vi "SavingToExistingCSV.vi"(9 "Numeric":dbl, 10 "all rows":dbl[][](array[numeric]), 11 "base path in":path) -> (1 "output array":dbl[][](array[numeric]), 2 "XY Graph 4":cluster{"array":dbl[], "array":dbl[]}, 3 "Last Rsh (Ohm)":dbl, 4 "appended array":dbl[](array[numeric]))   [LabVIEW 2017]
uses:
  <vilib>/Utility/file.llb/Read Delimited Spreadsheet (DBL).vi
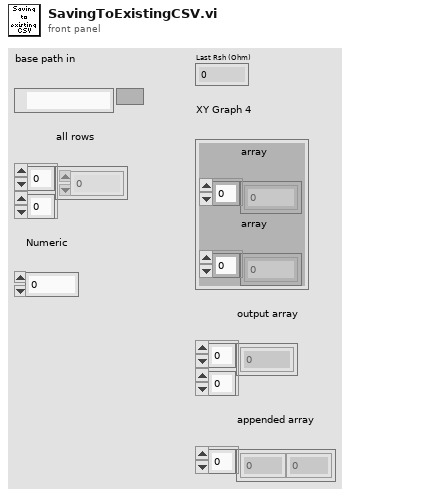
[diagram p1: front panel]
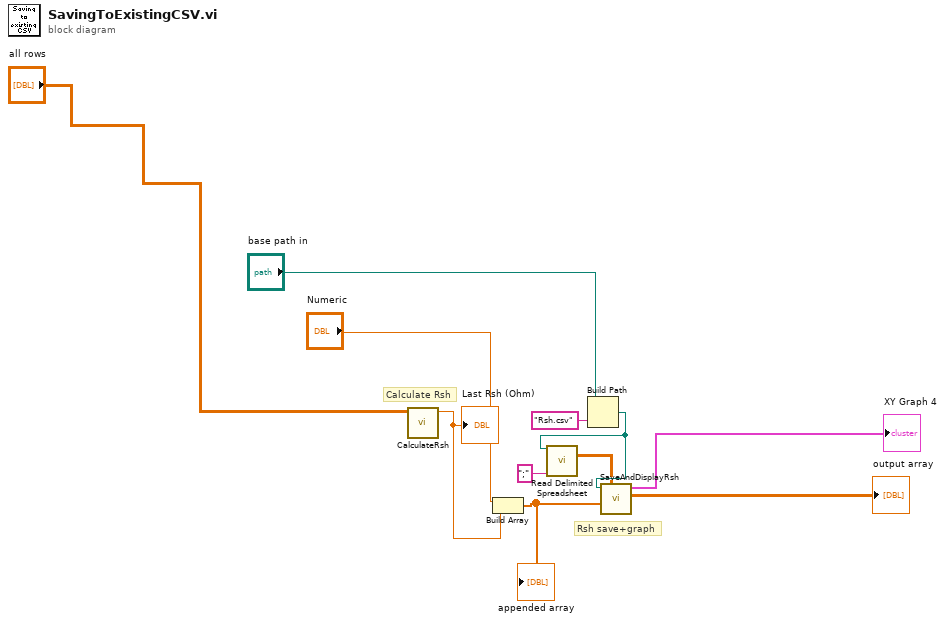
[diagram p0: block diagram]
diagram:
  # "Rsh save+graph"
  # "Calculate Rsh"
  n1 = call "CalculateRsh.vi"("Array"="all rows") -> ("Rsh (Ohm)"=w1:dbl)  [unwired: 10 in]
  "Last Rsh (Ohm)" <- w1
  n2 = Build Array("Numeric", w1) -> (w2:dbl[])
  "appended array" <- w2
  n3 = Build Path(base path="base path in", name or relative path="Rsh.csv") -> (appended path=w7:path)
  n4 = call-poly <vilib>:"Read Delimited Spreadsheet.vi"("file path (dialog if empty)"=w7, "delimiter (\\t)"=";" ("delimiter (\\t)")) -> ("all rows"=w6:dbl[][])  [unwired: 8 in, 5 out]
  n5 = call "SaveAndDisplayRsh.vi"("Array"=w2, "array"=w6, "file path (csv write)"=w7) -> ("output array"=→"output array":dbl[][], "XY Graph 4"=→"XY Graph 4":cluster{"array":dbl[], "array":dbl[]})  [unwired: 7 in]
